vi "rs3 Set All Advanced5.vi"(0 "Set Color Corr":bool=TRUE, 1 "Depth Presets":T2(ring), 2 "Color Presets":T1(ring), 7 "error in (no error)":errorcluster, 8 "device in":u64=370866768, 10 "ST_CensusEnable":cluster{"uDiameter":u32, "vDiameter":u32}={"uDiameter"=9, "vDiameter"=9}, 12 "ST_AE_Control":cluster{"meanIntensitySetpoint":u32}={"meanIntensitySetpoint"=400}, 16 "Depth Table":T3={"depthUnits, um"=1000, "depthClampMin"=0, "depthClampMax"=65535, "disparityMultiplier"=0, "disparityShift"=0}, 17 "ST RAU vector":T9={"minWest"=1, "minEast"=1, "minWEsum"=1, "minNorth"=1, "minSouth"=1, "minNSSum"=1, "uStrink"=1, "vShrink"=1}, 19 "ST Color Control":T8, 20 "depth control":T4={"plusIncrement"=10, "MinusDecrement"=10, "deepSeaMedianThreshold"=528, "scoreThreshA"=10, "scoreThreshB"=1023, "textureDifferenceThreshold"=0, "textureCountThreshold"=0, "deepSeaSecondPeakThreshold"=27, "deepSeaNeighborThreshold"=20, "IrAgreeThreshold"=70}, 21 "STColorCorrection":T11={"colorCorrection 1"=0.54785156, "colorCorrection 2"=0.32910156, "colorCorrection 3"=0.8222656, "colorCorrection 4"=0.109375, "colorCorrection 5"=-0.40527344, "colorCorrection 6"=-1.5253906, "colorCorrection 7"=0.95703125, "colorCorrection 8"=0.89160156, "colorCorrection 9"=0.7675781, "colorCorrection 10"=-0.4794922, "colorCorrection 11"=0.047851562, "colorCorrection 12"=-0.2705078}, 22 "HDAD":T12={"lambdaCensus"=26.0, "lambdaAD"=2100.0, "ignoreSAD"=0}, 23 "ST RSM":T10={"rsmBypass"=0, "diffThresh"=7.0, "sloRauDiffThresh"=3.0, "removeThresh"=33}, 24 "ST SLO Penalty":T5={"sloK1Penalty"=44, "sloK2Penalty"=502, "sloK1PenaltyMod1"=23, "sloK2PenaltyMod1"=237, "sloK1PenaltyMod2"=219, "sloK2PenaltyMod2"=113}, 25 "ST SLO Threshold":T6={"SLOdiffThresholdRed"=300, "SLODiffThresholdGreen"=300, "SLODiffThresholdBlue"=300}, 26 "ST Rau Threshold":T7={"rauDiffThresholdRed"=600, "rauDiffThresholdGreen"=600, "rauDiffThresholdBlue"=600}) -> (14 "Set advanced error":string, 18 "Dev out":u64=370866768, 27 "error out":errorcluster)   [LabVIEW 2018, in "libRealSense3.lvlib"]
doc: "The RealSense D4xx cameras are based on a stereo algorithm that has been accelerated as a fixed-function inside an ASIC. There are many parameters that affect the calculation of the depth. The basic task is to solve the correspondance problem - i.e. figure out which patches in the left image match up to those in the right image by doing a search along an epipolar line (x-axis). The x-axis difference for each object point is known as the disparity. \n\nIn general depth can be estimated for most points in the scene, but some points will have a very low confidence because 1. they are may be occluded (not seen by both imagers), or 2. have very little texture on them which will lead to an ambiquity (ex. when looking at a completely uniform white wall it, there are no best correspondances).\n\nThis VI allows you to set the many parameters that affect the algorith, as well as the color reproduction. \nNote that the color correction matrix will NOT have any effect on the depth calculations."
uses:
  libRealSense3.lvlib
panel:
  # "RS3 Set All Advanced 5"
  # "(C) 2017 Intel Corp.,  AGJ"
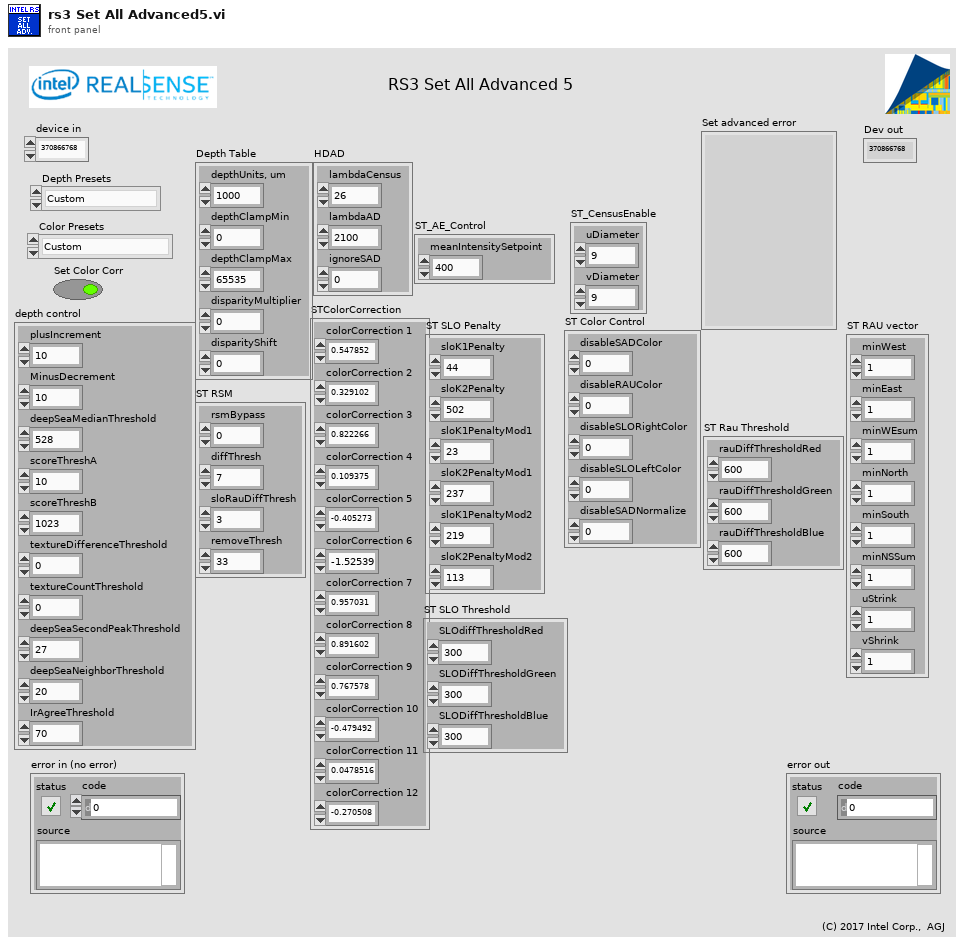
[diagram p1: front panel]
types:
  T1 = enum16{"Custom", "RS400 (DS5p)", "RS400 (DS5p) 2", "RS400 (DS5p) 3", "RS400 (DS5p) 4", "RS400 (DS5p) 5", "RS410 (DS5a)", "RS410 (DS5a) 2", "DS410 (DS5a) 3", "DS410 (DS5a) 4", "DS410+IR", "DS5LR", "DS5LR-2", "DS5LR no pattern", "RS410 Remove IR", "RS410 Remove IR 2", "DS5micro", "D435"}
  T2 = enum16{"Custom", "Original", "New Depth 1", "New Depth 2", "Depth Active 1", "Active 3D Scan", "Active Short A", "Active Short C", "Face", "Face2", "Best Box", "High Density", "Medium Density", "High Accuracy", "Hand", "Short Range", "Flat wall", "Load .JSON", "Load .JSON2"}
  T3 = cluster{"depthUnits, um":u32, "depthClampMin":u32, "depthClampMax":u32, "disparityMultiplier":u32, "disparityShift":u32}
  T4 = cluster{"plusIncrement":u32, "MinusDecrement":u32, "deepSeaMedianThreshold":u32, "scoreThreshA":u32, "scoreThreshB":u32, "textureDifferenceThreshold":u32, "textureCountThreshold":u32, "deepSeaSecondPeakThreshold":u32, "deepSeaNeighborThreshold":u32, "IrAgreeThreshold":u32}
  T5 = cluster{"sloK1Penalty":u32, "sloK2Penalty":u32, "sloK1PenaltyMod1":u32, "sloK2PenaltyMod1":u32, "sloK1PenaltyMod2":u32, "sloK2PenaltyMod2":u32}
  T6 = cluster{"SLOdiffThresholdRed":u32, "SLODiffThresholdGreen":u32, "SLODiffThresholdBlue":u32}
  T7 = cluster{"rauDiffThresholdRed":u32, "rauDiffThresholdGreen":u32, "rauDiffThresholdBlue":u32}
  T8 = cluster{"disableSADColor":u32, "disableRAUColor":u32, "disableSLORightColor":u32, "disableSLOLeftColor":u32, "disableSADNormalize":u32}
  T9 = cluster{"minWest":u32, "minEast":u32, "minWEsum":u32, "minNorth":u32, "minSouth":u32, "minNSSum":u32, "uStrink":u32, "vShrink":u32}
  T10 = cluster{"rsmBypass":u32, "diffThresh":sgl, "sloRauDiffThresh":sgl, "removeThresh":u32}
  T11 = cluster{"colorCorrection 1":sgl, "colorCorrection 2":sgl, "colorCorrection 3":sgl, "colorCorrection 4":sgl, "colorCorrection 5":sgl, "colorCorrection 6":sgl, "colorCorrection 7":sgl, "colorCorrection 8":sgl, "colorCorrection 9":sgl, "colorCorrection 10":sgl, "colorCorrection 11":sgl, "colorCorrection 12":sgl}
  T12 = cluster{"lambdaCensus":sgl, "lambdaAD":sgl, "ignoreSAD":u32}
  T13 = cluster{"rsmBypass (56)":u32, "diffThresh (57)":sgl, "sloRauDiffThresh(58)":sgl, "removeThresh(59)":u32}
  T14 = cluster{"depth control":cluster{"plusIncrement":u32, "MinusDecrement":u32, "deepSeaMedianThreshold":u32, "scoreThreshA":u32, "scoreThreshB":u32, "textureDifferenceThreshold":u32, "textureCountThreshold":u32, "deepSeaSecondPeakThreshold":u32, "deepSeaNeighborThreshold":u32, "IrAgreeThreshold":u32}, "STColorCorrection output":cluster{"colorCorrection 1":sgl, "colorCorrection 2":sgl, "colorCorrection 3":sgl, "colorCorrection 4":sgl, "colorCorrection 5":sgl, "colorCorrection 6":sgl, "colorCorrection 7":sgl, "colorCorrection 8":sgl, "colorCorrection 9":sgl, "colorCorrection 10":sgl, "colorCorrection 11":sgl, "colorCorrection 12":sgl}, "HDAD":cluster{"lambdaCensus":sgl, "lambdaAD":sgl, "ignoreSAD":u32}, "ST RSM":cluster{"rsmBypass":u32, "diffThresh":sgl, "sloRauDiffThresh":sgl, "removeThresh":u32}, "ST SLO Penalty":cluster{"sloK1Penalty":u32, "sloK2Penalty":u32, "sloK1PenaltyMod1":u32, "sloK2PenaltyMod1":u32, "sloK1PenaltyMod2":u32, "sloK2PenaltyMod2":u32}, "ST SLO Threshold":cluster{"SLOdiffThresholdRed":u32, "SLODiffThresholdGreen":u32, "SLODiffThresholdBlue":u32}, "ST Rau Threshold":cluster{"rauDiffThresholdRed":u32, "rauDiffThresholdGreen":u32, "rauDiffThresholdBlue":u32}, "ST Color Control":cluster{"disableSADColor":u32, "disableRAUColor":u32, "disableSLORightColor":u32, "disableSLOLeftColor":u32, "disableSADNormalize":u32}, "ST RAU vector":cluster{"minWest":u32, "minEast":u32, "minWEsum":u32, "minNorth":u32, "minSouth":u32, "minNSSum":u32, "uStrink":u32, "vShrink":u32}, "Depth Table":cluster{"depthUnits, um":u32, "depthClampMin":u32, "depthClampMax":u32, "disparityMultiplier":u32, "disparityShift":u32}, "ST_AE_Control":cluster{"meanIntensitySetpoint":u32}, "ST_CensusEnable":cluster{"uDiameter":u32, "vDiameter":u32}}
  T15 = cluster{"depthUnits, um":u32, "depthClampMin":u32, "depthClampMax":u32, "disparityMultiplier":u32, "disparityShift(0-127)":u32}
  T16 = cluster{"minWest (60)":u32, "minEast (61)":u32, "minWEsum (62)":u32, "minNorth (63)":u32, "minSouth (64)":u32, "minNSSum(65)":u32, "uStrink (66)":u32, "vShrink (67)":u32}
  T17 = cluster{"rauDiffThreshRed(73)":u32, "rauDiffThreshGreen(74)":u32, "rauDiffThreshBlue(75)":u32}
  T18 = cluster{"sloK1Penalty (79)":u32, "sloK2Penalty (80)":u32, "sloK1PenaltyMod1(81)":u32, "sloK2PenaltyMod1(82)":u32, "sloK1PenaltyMod2(83)":u32, "sloK2PenaltyMod2(84)":u32}
  T19 = cluster{"SLOdiffThreshRed(76)":u32, "SLODiffThreshGreen(77)":u32, "SLODiffThreshBlue(78)":u32}
  T20 = cluster{"disableSADColor(68)":u32, "disableRAUColor(69)":u32, "disableSLORightColor(70)":u32, "disableSLOLeftColor(71)":u32, "disableSADNormalize(72)":u32}
  T21 = cluster{"plusIncrement (47)":u32, "MinusDecrement (46)":u32, "deepSeaMedianThreshold (48)":u32, "scoreThreshA(49)":u32, "scoreThreshB (50)":u32, "textureDifferenceThreshold (52)":u32, "textureCountThreshold (51)":u32, "deepSea2ndPeakThresh.(53)":u32, "deepSeaNeighborThresh.(54)":u32, "LRAgreeThreshold (55)":u32}
  T22 = cluster{"plusIncrement (47)":u32, "MinusDecrement (46)":u32, "deepSeaMedianThreshold (48)":u32, "scoreThreshA(49)":u32, "scoreThreshB (50)":u32, "textureDifferenceThreshold (52)":u32, "textureCountThreshold (51)":u32, "deepSea2ndPeakThresh.(53)":u32, "deepSeaNeighborThresh.(54)":u32, "IrAgreeThreshold (55)":u32}
  T23 = cluster{"DS5p- 1":sgl, "colorCorrection 2":sgl, "colorCorrection 3":sgl, "colorCorrection 4":sgl, "colorCorrection 5":sgl, "colorCorrection 6":sgl, "colorCorrection 7":sgl, "colorCorrection 8":sgl, "colorCorrection 9":sgl, "colorCorrection 10":sgl, "colorCorrection 11":sgl, "colorCorrection 12":sgl}
  T24 = cluster{"Color 0":dbl, "Color 1":dbl, "Color 2":dbl, "Color 3":dbl, "Color 4":dbl, "Color 5":dbl, "Color 6":dbl, "Color 7":dbl, "Color 8":dbl, "Color 9":dbl, "Color 10":dbl, "Color 11":dbl}
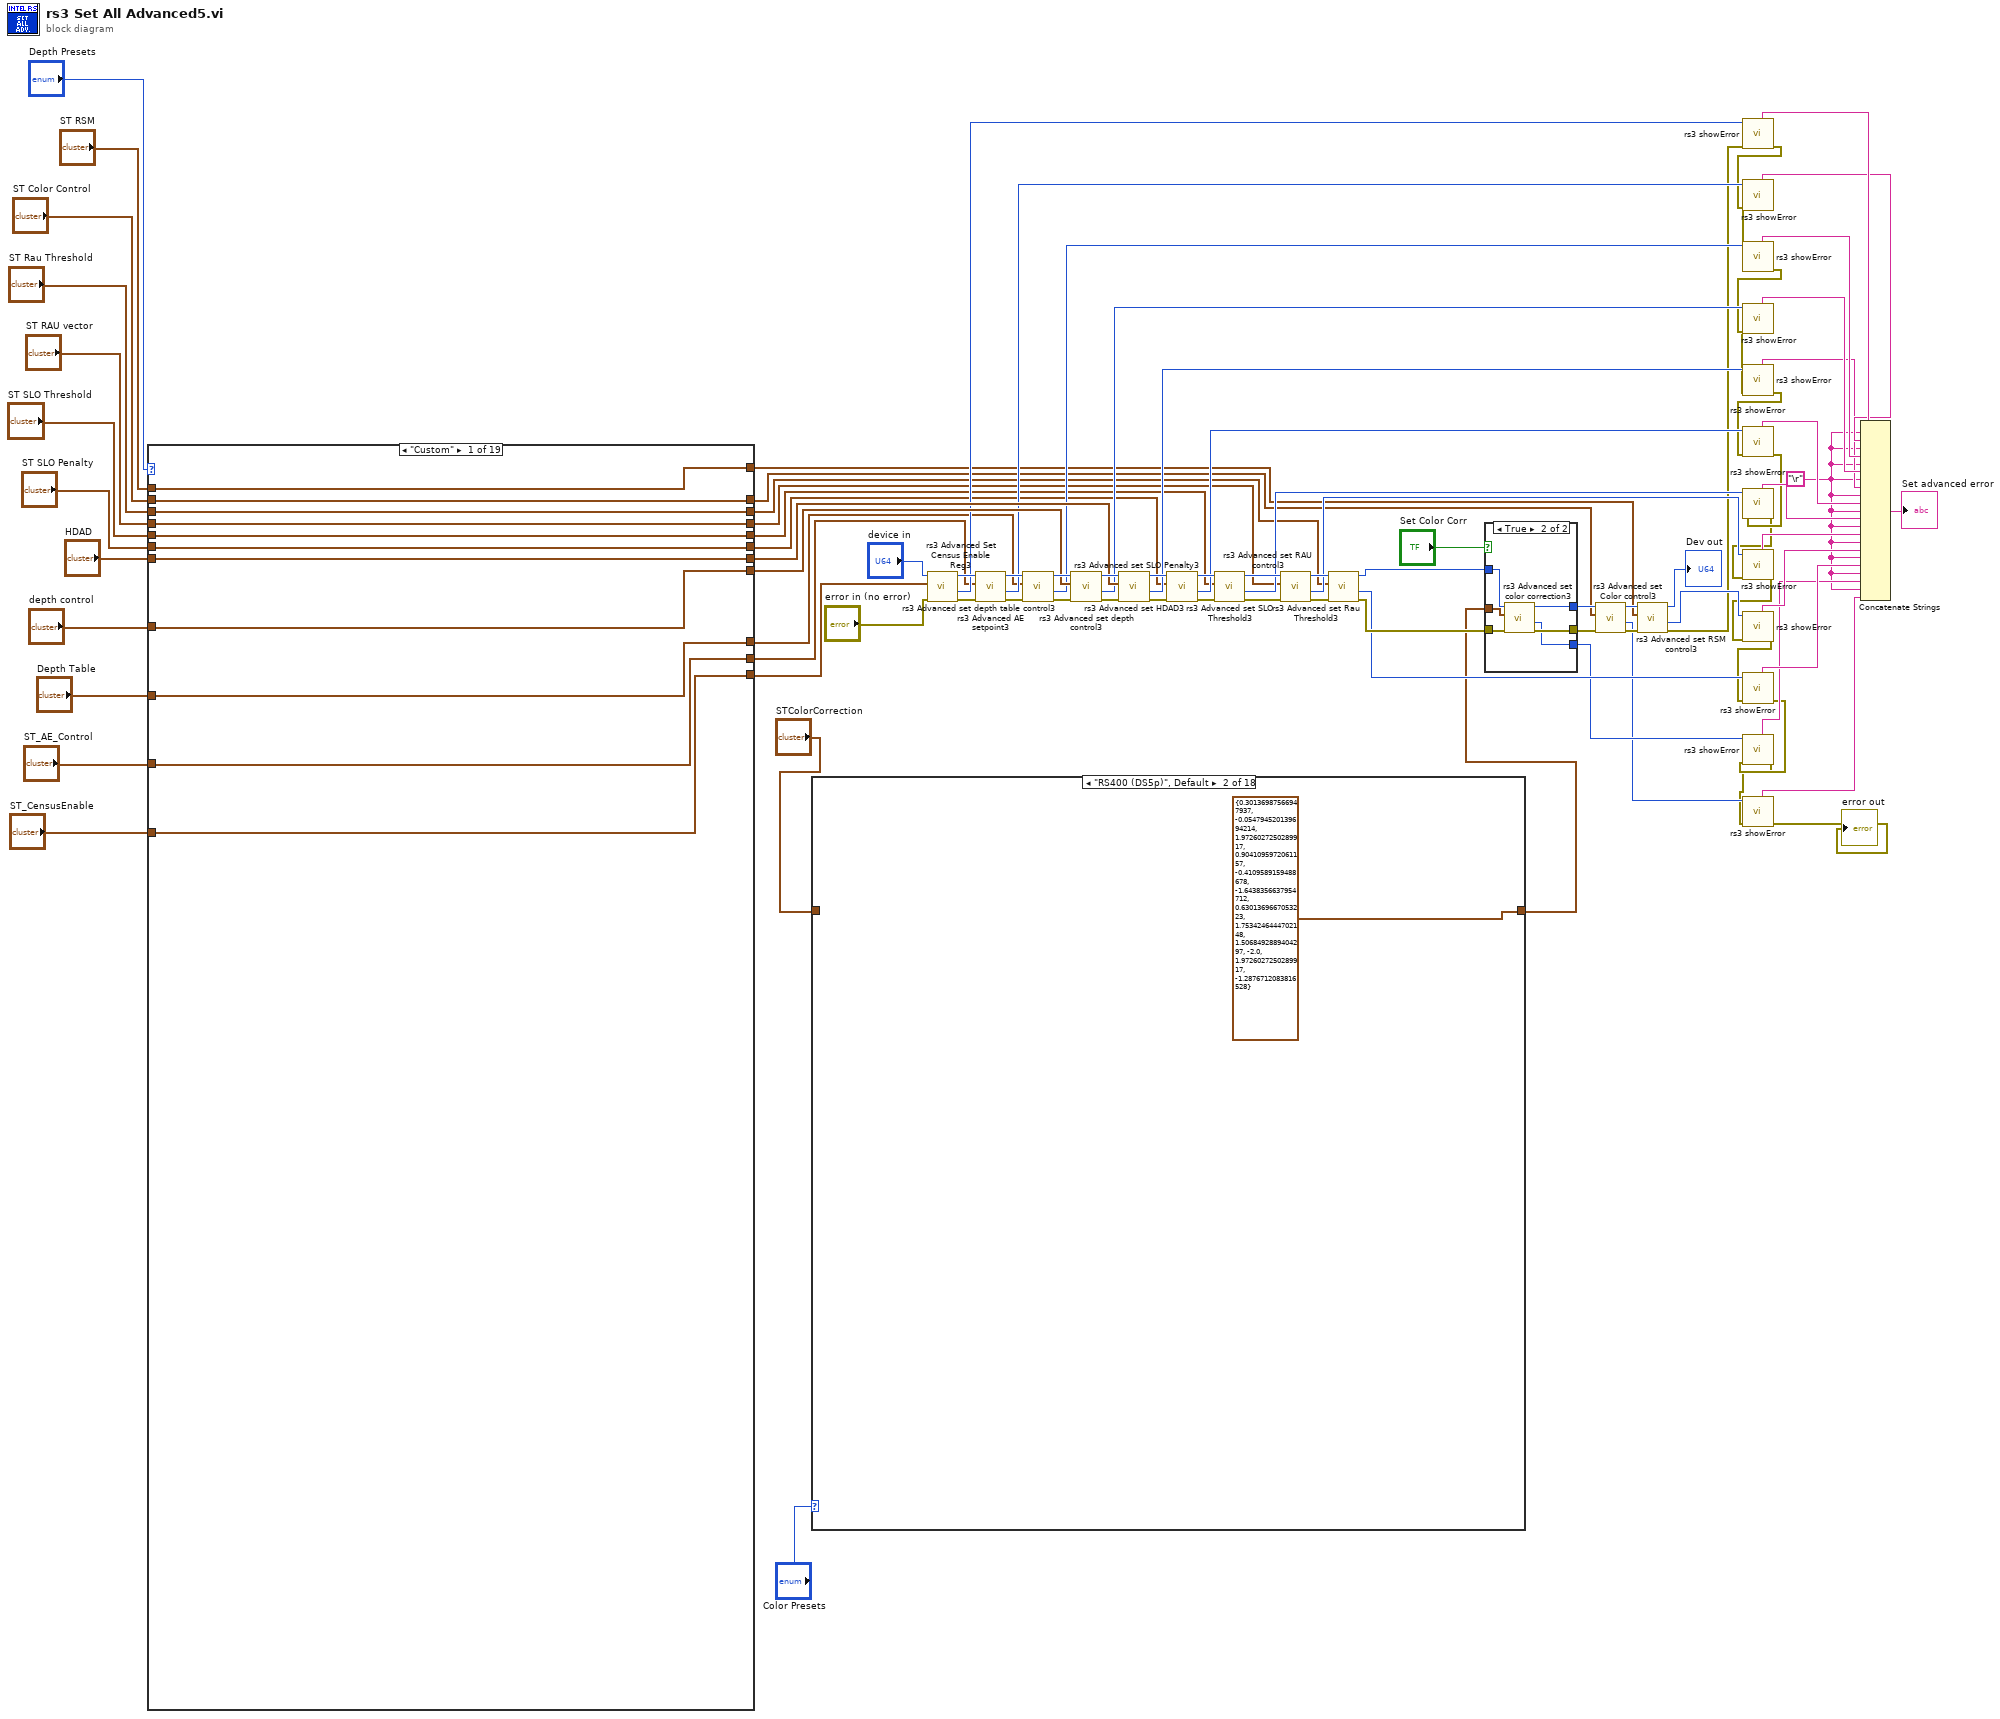
[diagram p0: block diagram]
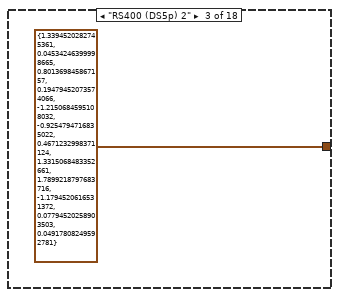
[diagram p3: hidden frame]
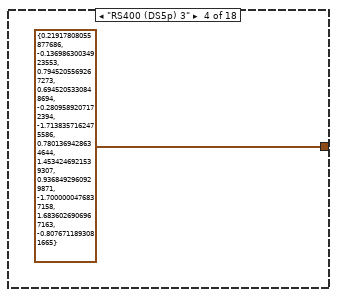
[diagram p4: hidden frame]
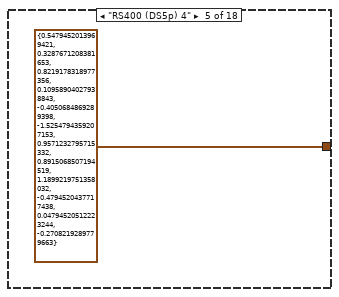
[diagram p5: hidden frame]
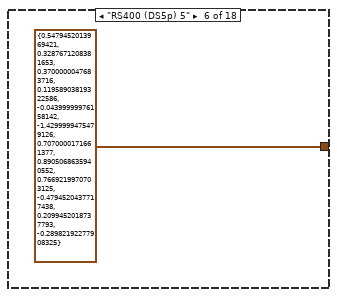
[diagram p6: hidden frame]
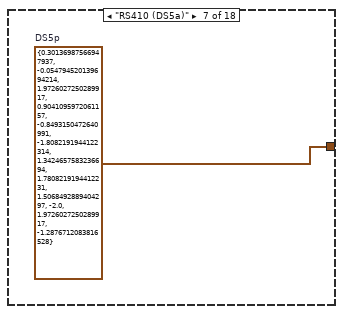
[diagram p7: hidden frame]
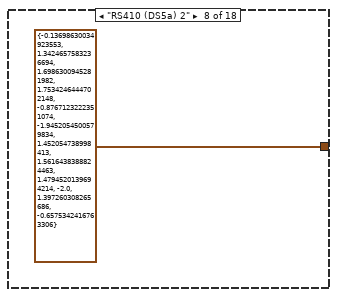
[diagram p8: hidden frame]
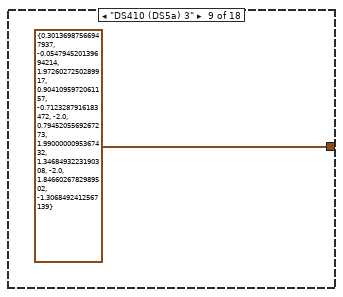
[diagram p9: hidden frame]
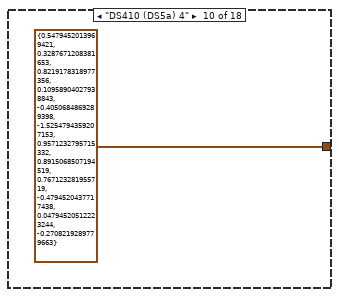
[diagram p10: hidden frame]
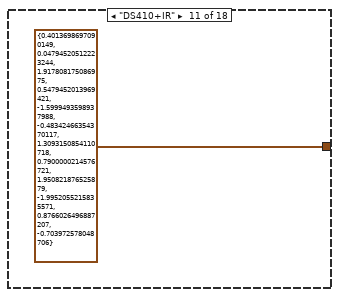
[diagram p11: hidden frame]
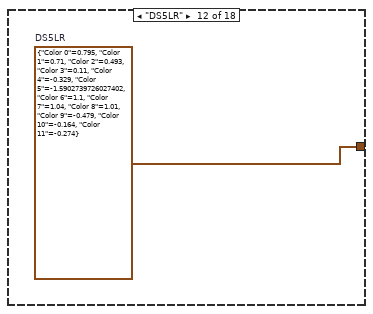
[diagram p12: hidden frame]
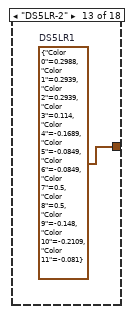
[diagram p13: hidden frame]
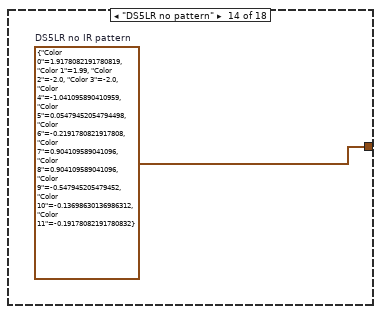
[diagram p14: hidden frame]
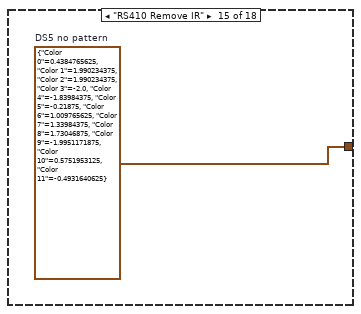
[diagram p15: hidden frame]
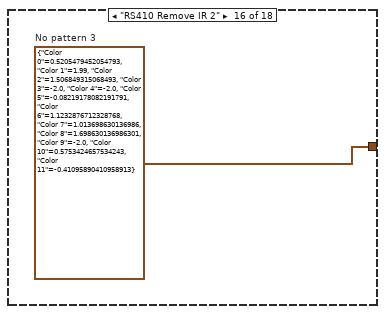
[diagram p16: hidden frame]
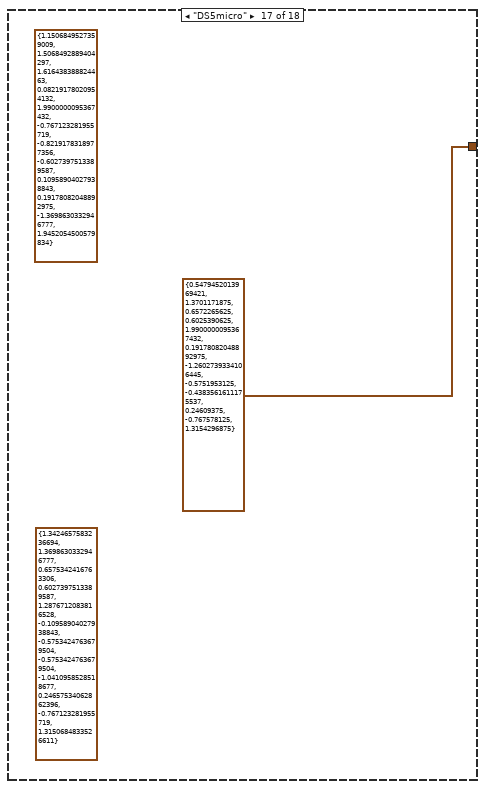
[diagram p17: hidden frame]
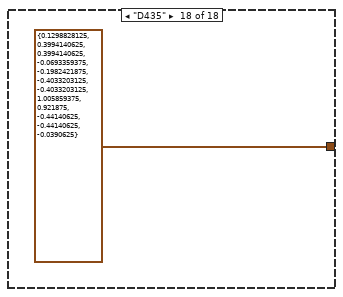
[diagram p18: hidden frame]
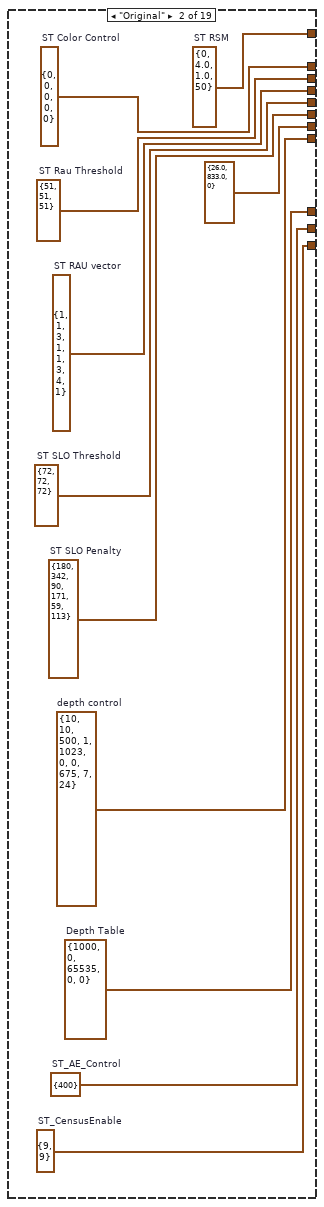
[diagram p19: hidden frame]
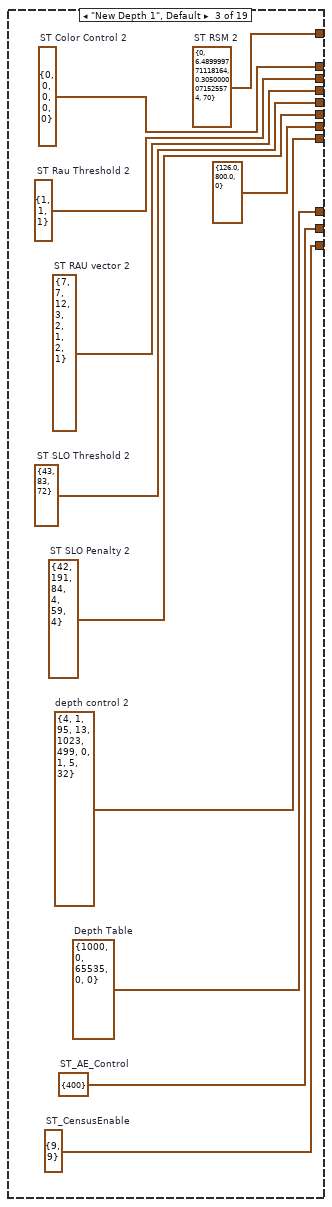
[diagram p20: hidden frame]
diagram:
  w36 = "\r"
  n1 = case shown="\"Custom\"" "Depth Presets" {
    tunnel: [w102 w112 w124 w135 w146 w150 w161 w172 w188 w198 w209 w216 w229 w241 w253 w265 w277 w292 w306] -> w63
    tunnel: [w96 w111 w123 w134 w145 T13 {"rsmBypass (56)"=0, "diffThresh (57)"=1.0367311, "sloRauDiffThresh(58)"=151.0, "removeThresh(59)"=1} ("ST RSM 2") w168 w179 w190 w195 w206 w221 w234 w246 w258 w270 w282 w294 w308] -> w25
    tunnel: [w97 w106 w122 w133 w144 w157 w167 w178 w189 w196 w207 w223 w236 w248 w260 w272 w284 w291 w305] -> w27
    tunnel: [w98 w107 w121 w132 w143 w156 w166 w177 w186 w197 w208 w219 w232 w244 w256 w268 w280 w295 w309] -> w28
    tunnel: [w95 w110 w120 w131 w142 w155 w165 w176 w185 w199 w210 w215 w228 w240 w252 w264 w276 w298 w312] -> w23
    tunnel: [w99 w109 w119 w130 w141 w154 w164 w175 w183 w200 w211 w214 w227 w239 w251 w263 w275 w297 w311] -> w30
    tunnel: [w100 w108 w118 w129 w140 w153 w163 w174 w187 w201 w212 w213 w226 w238 w250 w262 w274 w296 w310] -> w33
    tunnel: [w101 T12 {"lambdaCensus"=26.0, "lambdaAD"=833.0, "ignoreSAD"=0} ("HDAD 2") T12 {"lambdaCensus"=126.0, "lambdaAD"=800.0, "ignoreSAD"=0} ("HDAD 2") T12 {"lambdaCensus"=200.0, "lambdaAD"=1900.0, "ignoreSAD"=0} ("HDAD 2") T12 {"lambdaCensus"=216.0, "lambdaAD"=1400.0, "ignoreSAD"=0} ("HDAD 2") T12 {"lambdaCensus"=26.0, "lambdaAD"=833.0, "ignoreSAD"=0} ("HDAD 2") T12 {"lambdaCensus"=100.0, "lambdaAD"=1600.0, "ignoreSAD"=0} ("HDAD 2") w173 w184 T12 {"lambdaCensus"=26.0, "lambdaAD"=2100.0, "ignoreSAD"=0} ("HDAD*") T12 {"lambdaCensus"=15.0, "lambdaAD"=618.0, "ignoreSAD"=0} ("HDAD*") w222 w235 w247 w259 w271 w283 w293 w307] -> w61
    tunnel: [w93 w103 w114 w125 w136 w147 w158 w170 w180 w191 w202 w217 w230 w242 w254 w266 w278 w285 w301] -> w19
    tunnel: [w94 w104 w115 w126 w137 w148 w159 w169 w181 w192 w203 w218 w231 w243 w255 w267 w279 w286 w300] -> w21
    tunnel: [w92 w105 w116 w127 w138 w149 w160 w171 w182 w193 w204 w220 w233 w245 w257 w269 w281 w287 w299] -> w17
    tunnel: "depth control" -> [w102 _ _ _ _ _ _ _ _ _ _ _ _ _ _ _ _ _ _]
    tunnel: "HDAD" -> [w101 _ _ _ _ _ _ _ _ _ _ _ _ _ _ _ _ _ _]
    tunnel: "ST SLO Penalty" -> [w100 _ _ _ _ _ _ _ _ _ _ _ _ _ _ _ _ _ _]
    tunnel: "ST SLO Threshold" -> [w99 _ _ _ _ _ _ _ _ _ _ _ _ _ _ _ _ _ _]
    tunnel: "ST RAU vector" -> [w97 _ _ _ _ _ _ _ _ _ _ _ _ _ _ _ _ _ _]
    tunnel: "ST Rau Threshold" -> [w98 _ _ _ _ _ _ _ _ _ _ _ _ _ _ _ _ _ _]
    tunnel: "ST RSM" -> [w96 _ _ _ _ _ _ _ _ _ _ _ _ _ _ _ _ _ _]
    tunnel: "ST Color Control" -> [w95 _ _ _ _ _ _ _ _ _ _ _ _ _ _ _ _ _ _]
    tunnel: "ST_CensusEnable" -> [w94 _ _ _ _ _ _ _ _ _ _ _ _ _ _ _ _ _ _]
    tunnel: "ST_AE_Control" -> [w93 _ _ _ _ _ _ _ _ _ _ _ _ _ _ _ _ _ _]
    tunnel: "Depth Table" -> [w92 _ _ _ _ _ _ _ _ _ _ _ _ _ _ _ _ _ _]
    frame "Custom" {
    }
    frame "Original" {
      w104 = cluster{"uDiameter":u32, "vDiameter":u32} {"uDiameter"=9, "vDiameter"=9}  # ST_CensusEnable
      w105 = T15 {"depthUnits, um"=1000, "depthClampMin"=0, "depthClampMax"=65535, "disparityMultiplier"=0, "disparityShift(0-127)"=0}  # Depth Table
      w103 = cluster{"meanIntensitySetpoint":u32} {"meanIntensitySetpoint"=400}  # ST_AE_Control
      w106 = T16 {"minWest (60)"=1, "minEast (61)"=1, "minWEsum (62)"=3, "minNorth (63)"=1, "minSouth (64)"=1, "minNSSum(65)"=3, "uStrink (66)"=4, "vShrink (67)"=1}  # ST RAU vector
      w107 = T17 {"rauDiffThreshRed(73)"=51, "rauDiffThreshGreen(74)"=51, "rauDiffThreshBlue(75)"=51}  # ST Rau Threshold
      w108 = T18 {"sloK1Penalty (79)"=180, "sloK2Penalty (80)"=342, "sloK1PenaltyMod1(81)"=90, "sloK2PenaltyMod1(82)"=171, "sloK1PenaltyMod2(83)"=59, "sloK2PenaltyMod2(84)"=113}  # ST SLO Penalty
      w109 = T19 {"SLOdiffThreshRed(76)"=72, "SLODiffThreshGreen(77)"=72, "SLODiffThreshBlue(78)"=72}  # ST SLO Threshold
      w110 = T20 {"disableSADColor(68)"=0, "disableRAUColor(69)"=0, "disableSLORightColor(70)"=0, "disableSLOLeftColor(71)"=0, "disableSADNormalize(72)"=0}  # ST Color Control
      w111 = T13 {"rsmBypass (56)"=0, "diffThresh (57)"=4.0, "sloRauDiffThresh(58)"=1.0, "removeThresh(59)"=50}  # ST RSM
      w112 = T21 {"plusIncrement (47)"=10, "MinusDecrement (46)"=10, "deepSeaMedianThreshold (48)"=500, "scoreThreshA(49)"=1, "scoreThreshB (50)"=1023, "textureDifferenceThreshold (52)"=0, "textureCountThreshold (51)"=0, "deepSea2ndPeakThresh.(53)"=675, "deepSeaNeighborThresh.(54)"=7, "LRAgreeThreshold (55)"=24}  # depth control
    }
    frame "New Depth 1", Default {
      w115 = cluster{"uDiameter":u32, "vDiameter":u32} {"uDiameter"=9, "vDiameter"=9}  # ST_CensusEnable
      w116 = T15 {"depthUnits, um"=1000, "depthClampMin"=0, "depthClampMax"=65535, "disparityMultiplier"=0, "disparityShift(0-127)"=0}  # Depth Table
      w114 = cluster{"meanIntensitySetpoint":u32} {"meanIntensitySetpoint"=400}  # ST_AE_Control
      w118 = T18 {"sloK1Penalty (79)"=42, "sloK2Penalty (80)"=191, "sloK1PenaltyMod1(81)"=84, "sloK2PenaltyMod1(82)"=4, "sloK1PenaltyMod2(83)"=59, "sloK2PenaltyMod2(84)"=4}  # ST SLO Penalty 2
      w119 = T19 {"SLOdiffThreshRed(76)"=43, "SLODiffThreshGreen(77)"=83, "SLODiffThreshBlue(78)"=72}  # ST SLO Threshold 2
      w120 = T20 {"disableSADColor(68)"=0, "disableRAUColor(69)"=0, "disableSLORightColor(70)"=0, "disableSLOLeftColor(71)"=0, "disableSADNormalize(72)"=0}  # ST Color Control 2
      w121 = T17 {"rauDiffThreshRed(73)"=1, "rauDiffThreshGreen(74)"=1, "rauDiffThreshBlue(75)"=1}  # ST Rau Threshold 2
      w122 = T16 {"minWest (60)"=7, "minEast (61)"=7, "minWEsum (62)"=12, "minNorth (63)"=3, "minSouth (64)"=2, "minNSSum(65)"=1, "uStrink (66)"=2, "vShrink (67)"=1}  # ST RAU vector 2
      w123 = T13 {"rsmBypass (56)"=0, "diffThresh (57)"=6.49, "sloRauDiffThresh(58)"=0.305, "removeThresh(59)"=70}  # ST RSM 2
      w124 = T22 {"plusIncrement (47)"=4, "MinusDecrement (46)"=1, "deepSeaMedianThreshold (48)"=95, "scoreThreshA(49)"=13, "scoreThreshB (50)"=1023, "textureDifferenceThreshold (52)"=499, "textureCountThreshold (51)"=0, "deepSea2ndPeakThresh.(53)"=1, "deepSeaNeighborThresh.(54)"=5, "IrAgreeThreshold (55)"=32}  # depth control 2
    }
    frame "New Depth 2" {
      w126 = cluster{"uDiameter":u32, "vDiameter":u32} {"uDiameter"=9, "vDiameter"=9}  # ST_CensusEnable
      w127 = T15 {"depthUnits, um"=1000, "depthClampMin"=0, "depthClampMax"=65535, "disparityMultiplier"=0, "disparityShift(0-127)"=0}  # Depth Table
      w125 = cluster{"meanIntensitySetpoint":u32} {"meanIntensitySetpoint"=400}  # ST_AE_Control
      w129 = T18 {"sloK1Penalty (79)"=42, "sloK2Penalty (80)"=191, "sloK1PenaltyMod1(81)"=84, "sloK2PenaltyMod1(82)"=4, "sloK1PenaltyMod2(83)"=59, "sloK2PenaltyMod2(84)"=4}  # ST SLO Penalty 2
      w130 = T19 {"SLOdiffThreshRed(76)"=100, "SLODiffThreshGreen(77)"=100, "SLODiffThreshBlue(78)"=100}  # ST SLO Threshold 2
      w131 = T20 {"disableSADColor(68)"=0, "disableRAUColor(69)"=0, "disableSLORightColor(70)"=0, "disableSLOLeftColor(71)"=0, "disableSADNormalize(72)"=0}  # ST Color Control 2
      w132 = T17 {"rauDiffThreshRed(73)"=50, "rauDiffThreshGreen(74)"=50, "rauDiffThreshBlue(75)"=50}  # ST Rau Threshold 2
      w133 = T16 {"minWest (60)"=1, "minEast (61)"=1, "minWEsum (62)"=9, "minNorth (63)"=3, "minSouth (64)"=2, "minNSSum(65)"=1, "uStrink (66)"=2, "vShrink (67)"=1}  # ST RAU vector 2
      w134 = T13 {"rsmBypass (56)"=0, "diffThresh (57)"=6.49, "sloRauDiffThresh(58)"=0.305, "removeThresh(59)"=50}  # ST RSM 2
      w135 = T22 {"plusIncrement (47)"=4, "MinusDecrement (46)"=1, "deepSeaMedianThreshold (48)"=95, "scoreThreshA(49)"=13, "scoreThreshB (50)"=1023, "textureDifferenceThreshold (52)"=499, "textureCountThreshold (51)"=0, "deepSea2ndPeakThresh.(53)"=1, "deepSeaNeighborThresh.(54)"=5, "IrAgreeThreshold (55)"=200}  # depth control 2
    }
    frame "Depth Active 1" {
      w137 = cluster{"uDiameter":u32, "vDiameter":u32} {"uDiameter"=9, "vDiameter"=9}  # ST_CensusEnable
      w138 = T15 {"depthUnits, um"=1000, "depthClampMin"=0, "depthClampMax"=65535, "disparityMultiplier"=0, "disparityShift(0-127)"=0}  # Depth Table
      w136 = cluster{"meanIntensitySetpoint":u32} {"meanIntensitySetpoint"=400}  # ST_AE_Control
      w140 = T18 {"sloK1Penalty (79)"=10, "sloK2Penalty (80)"=60, "sloK1PenaltyMod1(81)"=84, "sloK2PenaltyMod1(82)"=56, "sloK1PenaltyMod2(83)"=59, "sloK2PenaltyMod2(84)"=4}  # ST SLO Penalty 2
      w141 = T19 {"SLOdiffThreshRed(76)"=200, "SLODiffThreshGreen(77)"=200, "SLODiffThreshBlue(78)"=200}  # ST SLO Threshold 2
      w142 = T20 {"disableSADColor(68)"=0, "disableRAUColor(69)"=0, "disableSLORightColor(70)"=0, "disableSLOLeftColor(71)"=0, "disableSADNormalize(72)"=0}  # ST Color Control 2
      w143 = T17 {"rauDiffThreshRed(73)"=70, "rauDiffThreshGreen(74)"=70, "rauDiffThreshBlue(75)"=70}  # ST Rau Threshold 2
      w144 = T16 {"minWest (60)"=7, "minEast (61)"=7, "minWEsum (62)"=12, "minNorth (63)"=3, "minSouth (64)"=2, "minNSSum(65)"=1, "uStrink (66)"=2, "vShrink (67)"=1}  # ST RAU vector 2
      w145 = T13 {"rsmBypass (56)"=0, "diffThresh (57)"=6.49, "sloRauDiffThresh(58)"=0.305, "removeThresh(59)"=60}  # ST RSM 2
      w146 = T22 {"plusIncrement (47)"=4, "MinusDecrement (46)"=1, "deepSeaMedianThreshold (48)"=95, "scoreThreshA(49)"=13, "scoreThreshB (50)"=1023, "textureDifferenceThreshold (52)"=499, "textureCountThreshold (51)"=0, "deepSea2ndPeakThresh.(53)"=1, "deepSeaNeighborThresh.(54)"=5, "IrAgreeThreshold (55)"=82}  # depth control 2
    }
    frame "Active 3D Scan" {
      w148 = cluster{"uDiameter":u32, "vDiameter":u32} {"uDiameter"=9, "vDiameter"=9}  # ST_CensusEnable
      w149 = T15 {"depthUnits, um"=1000, "depthClampMin"=0, "depthClampMax"=65535, "disparityMultiplier"=0, "disparityShift(0-127)"=0}  # Depth Table
      w147 = cluster{"meanIntensitySetpoint":u32} {"meanIntensitySetpoint"=400}  # ST_AE_Control
      w150 = T22 {"plusIncrement (47)"=19, "MinusDecrement (46)"=4, "deepSeaMedianThreshold (48)"=554, "scoreThreshA(49)"=1, "scoreThreshB (50)"=632, "textureDifferenceThreshold (52)"=0, "textureCountThreshold (51)"=31, "deepSea2ndPeakThresh.(53)"=665, "deepSeaNeighborThresh.(54)"=126, "IrAgreeThreshold (55)"=11}  # depth control 2
      w153 = T18 {"sloK1Penalty (79)"=93, "sloK2Penalty (80)"=473, "sloK1PenaltyMod1(81)"=70, "sloK2PenaltyMod1(82)"=123, "sloK1PenaltyMod2(83)"=92, "sloK2PenaltyMod2(84)"=409}  # ST SLO Penalty 2
      w154 = T19 {"SLOdiffThreshRed(76)"=46, "SLODiffThreshGreen(77)"=442, "SLODiffThreshBlue(78)"=105}  # ST SLO Threshold 2
      w155 = T20 {"disableSADColor(68)"=0, "disableRAUColor(69)"=0, "disableSLORightColor(70)"=0, "disableSLOLeftColor(71)"=0, "disableSADNormalize(72)"=0}  # ST Color Control 2
      w156 = T17 {"rauDiffThreshRed(73)"=46, "rauDiffThreshGreen(74)"=442, "rauDiffThreshBlue(75)"=105}  # ST Rau Threshold 2
      w157 = T16 {"minWest (60)"=5, "minEast (61)"=7, "minWEsum (62)"=12, "minNorth (63)"=1, "minSouth (64)"=3, "minNSSum(65)"=7, "uStrink (66)"=4, "vShrink (67)"=1}  # ST RAU vector 2
    }
    frame "Active Short A" {
      w159 = cluster{"uDiameter":u32, "vDiameter":u32} {"uDiameter"=3, "vDiameter"=3}  # ST_CensusEnable
      w160 = T15 {"depthUnits, um"=200, "depthClampMin"=0, "depthClampMax"=65535, "disparityMultiplier"=0, "disparityShift(0-127)"=0}  # Depth Table
      w158 = cluster{"meanIntensitySetpoint":u32} {"meanIntensitySetpoint"=400}  # ST_AE_Control
      w161 = T22 {"plusIncrement (47)"=7, "MinusDecrement (46)"=1, "deepSeaMedianThreshold (48)"=140, "scoreThreshA(49)"=10, "scoreThreshB (50)"=1023, "textureDifferenceThreshold (52)"=499, "textureCountThreshold (51)"=0, "deepSea2ndPeakThresh.(53)"=1, "deepSeaNeighborThresh.(54)"=5, "IrAgreeThreshold (55)"=80}  # depth control 2
      w163 = T18 {"sloK1Penalty (79)"=5, "sloK2Penalty (80)"=30, "sloK1PenaltyMod1(81)"=11, "sloK2PenaltyMod1(82)"=50, "sloK1PenaltyMod2(83)"=56, "sloK2PenaltyMod2(84)"=15}  # ST SLO Penalty 2
      w164 = T19 {"SLOdiffThreshRed(76)"=200, "SLODiffThreshGreen(77)"=200, "SLODiffThreshBlue(78)"=200}  # ST SLO Threshold 2
      w165 = T20 {"disableSADColor(68)"=0, "disableRAUColor(69)"=0, "disableSLORightColor(70)"=0, "disableSLOLeftColor(71)"=0, "disableSADNormalize(72)"=0}  # ST Color Control 2
      w166 = T17 {"rauDiffThreshRed(73)"=200, "rauDiffThreshGreen(74)"=200, "rauDiffThreshBlue(75)"=200}  # ST Rau Threshold 2
      w167 = T16 {"minWest (60)"=3, "minEast (61)"=3, "minWEsum (62)"=13, "minNorth (63)"=1, "minSouth (64)"=1, "minNSSum(65)"=1, "uStrink (66)"=4, "vShrink (67)"=4}  # ST RAU vector 2
      w168 = T13 {"rsmBypass (56)"=0, "diffThresh (57)"=7.5, "sloRauDiffThresh(58)"=0.9, "removeThresh(59)"=72}  # ST RSM 2
    }
    frame "Active Short C" {
      w169 = cluster{"uDiameter":u32, "vDiameter":u32} {"uDiameter"=3, "vDiameter"=3}  # ST_CensusEnable
      w171 = T15 {"depthUnits, um"=200, "depthClampMin"=0, "depthClampMax"=65535, "disparityMultiplier"=0, "disparityShift(0-127)"=0}  # Depth Table
      w170 = cluster{"meanIntensitySetpoint":u32} {"meanIntensitySetpoint"=400}  # ST_AE_Control
      w172 = T22 {"plusIncrement (47)"=10, "MinusDecrement (46)"=10, "deepSeaMedianThreshold (48)"=415, "scoreThreshA(49)"=1, "scoreThreshB (50)"=1023, "textureDifferenceThreshold (52)"=0, "textureCountThreshold (51)"=14, "deepSea2ndPeakThresh.(53)"=56, "deepSeaNeighborThresh.(54)"=108, "IrAgreeThreshold (55)"=8}  # depth control 2
      w173 = T12 {"lambdaCensus"=26.0, "lambdaAD"=958.0, "ignoreSAD"=0}  # HDAD 2
      w174 = T18 {"sloK1Penalty (79)"=203, "sloK2Penalty (80)"=342, "sloK1PenaltyMod1(81)"=109, "sloK2PenaltyMod1(82)"=502, "sloK1PenaltyMod2(83)"=209, "sloK2PenaltyMod2(84)"=14}  # ST SLO Penalty 2
      w175 = T19 {"SLOdiffThreshRed(76)"=889, "SLODiffThreshGreen(77)"=69, "SLODiffThreshBlue(78)"=189}  # ST SLO Threshold 2
      w176 = T20 {"disableSADColor(68)"=0, "disableRAUColor(69)"=0, "disableSLORightColor(70)"=0, "disableSLOLeftColor(71)"=0, "disableSADNormalize(72)"=0}  # ST Color Control 2
      w177 = T17 {"rauDiffThreshRed(73)"=298, "rauDiffThreshGreen(74)"=95, "rauDiffThreshBlue(75)"=675}  # ST Rau Threshold 2
      w178 = T16 {"minWest (60)"=1, "minEast (61)"=1, "minWEsum (62)"=3, "minNorth (63)"=1, "minSouth (64)"=1, "minNSSum(65)"=3, "uStrink (66)"=3, "vShrink (67)"=1}  # ST RAU vector 2
      w179 = T13 {"rsmBypass (56)"=0, "diffThresh (57)"=5.386, "sloRauDiffThresh(58)"=0.9687, "removeThresh(59)"=88}  # ST RSM 2
    }
    frame "Face" {
      w181 = cluster{"uDiameter":u32, "vDiameter":u32} {"uDiameter"=9, "vDiameter"=9}  # ST_CensusEnable
      w182 = T15 {"depthUnits, um"=1000, "depthClampMin"=0, "depthClampMax"=65535, "disparityMultiplier"=0, "disparityShift(0-127)"=0}  # Depth Table
      w180 = cluster{"meanIntensitySetpoint":u32} {"meanIntensitySetpoint"=800}  # ST_AE_Control
      w184 = T12 {"lambdaCensus"=26.0, "lambdaAD"=2100.0, "ignoreSAD"=0}  # HDAD*
      w183 = T19 {"SLOdiffThreshRed(76)"=300, "SLODiffThreshGreen(77)"=300, "SLODiffThreshBlue(78)"=300}  # ST SLO Threshold
      w185 = T20 {"disableSADColor(68)"=0, "disableRAUColor(69)"=0, "disableSLORightColor(70)"=0, "disableSLOLeftColor(71)"=0, "disableSADNormalize(72)"=0}  # ST Color Control
      w186 = T17 {"rauDiffThreshRed(73)"=600, "rauDiffThreshGreen(74)"=600, "rauDiffThreshBlue(75)"=600}  # ST Rau Threshold
      w187 = T18 {"sloK1Penalty (79)"=44, "sloK2Penalty (80)"=502, "sloK1PenaltyMod1(81)"=23, "sloK2PenaltyMod1(82)"=237, "sloK1PenaltyMod2(83)"=219, "sloK2PenaltyMod2(84)"=113}  # ST SLO Penalty
      w188 = T21 {"plusIncrement (47)"=10, "MinusDecrement (46)"=10, "deepSeaMedianThreshold (48)"=528, "scoreThreshA(49)"=10, "scoreThreshB (50)"=1023, "textureDifferenceThreshold (52)"=0, "textureCountThreshold (51)"=0, "deepSea2ndPeakThresh.(53)"=27, "deepSeaNeighborThresh.(54)"=20, "LRAgreeThreshold (55)"=70}  # depth control
      w189 = T16 {"minWest (60)"=1, "minEast (61)"=1, "minWEsum (62)"=1, "minNorth (63)"=1, "minSouth (64)"=1, "minNSSum(65)"=1, "uStrink (66)"=1, "vShrink (67)"=1}  # ST RAU vector
      w190 = T13 {"rsmBypass (56)"=0, "diffThresh (57)"=7.0, "sloRauDiffThresh(58)"=3.0, "removeThresh(59)"=33}  # ST RSM
    }
    frame "Face2" {
      w192 = cluster{"uDiameter":u32, "vDiameter":u32} {"uDiameter"=9, "vDiameter"=9}  # ST_CensusEnable
      w193 = T15 {"depthUnits, um"=1000, "depthClampMin"=0, "depthClampMax"=65535, "disparityMultiplier"=0, "disparityShift(0-127)"=0}  # Depth Table
      w191 = cluster{"meanIntensitySetpoint":u32} {"meanIntensitySetpoint"=800}  # ST_AE_Control
      w195 = T13 {"rsmBypass (56)"=0, "diffThresh (57)"=1.21875, "sloRauDiffThresh(58)"=0.28125, "removeThresh(59)"=83}  # ST RSM
      w196 = T16 {"minWest (60)"=3, "minEast (61)"=2, "minWEsum (62)"=7, "minNorth (63)"=1, "minSouth (64)"=3, "minNSSum(65)"=6, "uStrink (66)"=4, "vShrink (67)"=0}  # ST RAU vector
      w197 = T17 {"rauDiffThreshRed(73)"=18, "rauDiffThreshGreen(74)"=113, "rauDiffThreshBlue(75)"=586}  # ST Rau Threshold
      w198 = T21 {"plusIncrement (47)"=10, "MinusDecrement (46)"=10, "deepSeaMedianThreshold (48)"=528, "scoreThreshA(49)"=10, "scoreThreshB (50)"=1023, "textureDifferenceThreshold (52)"=0, "textureCountThreshold (51)"=0, "deepSea2ndPeakThresh.(53)"=27, "deepSeaNeighborThresh.(54)"=20, "LRAgreeThreshold (55)"=70}  # depth control
      w199 = T20 {"disableSADColor(68)"=0, "disableRAUColor(69)"=0, "disableSLORightColor(70)"=0, "disableSLOLeftColor(71)"=0, "disableSADNormalize(72)"=0}  # ST Color Control
      w200 = T19 {"SLOdiffThreshRed(76)"=279, "SLODiffThreshGreen(77)"=200, "SLODiffThreshBlue(78)"=8}  # ST SLO Threshold
      w201 = T18 {"sloK1Penalty (79)"=55, "sloK2Penalty (80)"=235, "sloK1PenaltyMod1(81)"=326, "sloK2PenaltyMod1(82)"=506, "sloK1PenaltyMod2(83)"=134, "sloK2PenaltyMod2(84)"=206}  # ST SLO Penalty
    }
    frame "Best Box" {
      w203 = cluster{"uDiameter":u32, "vDiameter":u32} {"uDiameter"=9, "vDiameter"=9}  # ST_CensusEnable
      w204 = T15 {"depthUnits, um"=1000, "depthClampMin"=0, "depthClampMax"=65535, "disparityMultiplier"=0, "disparityShift(0-127)"=0}  # Depth Table
      w202 = cluster{"meanIntensitySetpoint":u32} {"meanIntensitySetpoint"=400}  # ST_AE_Control
      w206 = T13 {"rsmBypass (56)"=0, "diffThresh (57)"=1.21875, "sloRauDiffThresh(58)"=0.28125, "removeThresh(59)"=83}  # ST RSM
      w207 = T16 {"minWest (60)"=3, "minEast (61)"=2, "minWEsum (62)"=7, "minNorth (63)"=1, "minSouth (64)"=3, "minNSSum(65)"=6, "uStrink (66)"=4, "vShrink (67)"=0}  # ST RAU vector
      w208 = T17 {"rauDiffThreshRed(73)"=18, "rauDiffThreshGreen(74)"=113, "rauDiffThreshBlue(75)"=586}  # ST Rau Threshold
      w209 = T21 {"plusIncrement (47)"=10, "MinusDecrement (46)"=10, "deepSeaMedianThreshold (48)"=528, "scoreThreshA(49)"=10, "scoreThreshB (50)"=1023, "textureDifferenceThreshold (52)"=0, "textureCountThreshold (51)"=0, "deepSea2ndPeakThresh.(53)"=27, "deepSeaNeighborThresh.(54)"=20, "LRAgreeThreshold (55)"=70}  # depth control
      w210 = T20 {"disableSADColor(68)"=0, "disableRAUColor(69)"=0, "disableSLORightColor(70)"=0, "disableSLOLeftColor(71)"=0, "disableSADNormalize(72)"=0}  # ST Color Control
      w211 = T19 {"SLOdiffThreshRed(76)"=279, "SLODiffThreshGreen(77)"=200, "SLODiffThreshBlue(78)"=8}  # ST SLO Threshold
      w212 = T18 {"sloK1Penalty (79)"=55, "sloK2Penalty (80)"=235, "sloK1PenaltyMod1(81)"=326, "sloK2PenaltyMod1(82)"=506, "sloK1PenaltyMod2(83)"=134, "sloK2PenaltyMod2(84)"=206}  # ST SLO Penalty
    }
    frame "High Density" {
      n2 = Unbundle By Name(T14 {"depth control"={"plusIncrement"=21, "MinusDecrement"=6, "deepSeaMedianThreshold"=789, "scoreThreshA"=96, "scoreThreshB"=1443, "textureDifferenceThreshold"=2466, "textureCountThreshold"=0, "deepSeaSecondPeakThreshold"=222, "deepSeaNeighborThreshold"=12, "IrAgreeThreshold"=18}, "STColorCorrection output"={"colorCorrection 1"=0.54785156, "colorCorrection 2"=0.32910156, "colorCorrection 3"=0.8222656, "colorCorrection 4"=0.109375, "colorCorrection 5"=-0.40527344, "colorCorrection 6"=-1.5253906, "colorCorrection 7"=0.95703125, "colorCorrection 8"=0.89160156, "colorCorrection 9"=0.7675781, "colorCorrection 10"=-0.4794922, "colorCorrection 11"=0.047851562, "colorCorrection 12"=-0.2705078}, "HDAD"={"lambdaCensus"=15.0, "lambdaAD"=618.0, "ignoreSAD"=0}, "ST RSM"={"rsmBypass"=0, "diffThresh"=1.21875, "sloRauDiffThresh"=0.28125, "removeThresh"=82}, "ST SLO Penalty"={"sloK1Penalty"=55, "sloK2Penalty"=235, "sloK1PenaltyMod1"=326, "sloK2PenaltyMod1"=506, "sloK1PenaltyMod2"=134, "sloK2PenaltyMod2"=206}, "ST SLO Threshold"={"SLOdiffThresholdRed"=279, "SLODiffThresholdGreen"=200, "SLODiffThresholdBlue"=8}, "ST Rau Threshold"={"rauDiffThresholdRed"=18, "rauDiffThresholdGreen"=585, "rauDiffThresholdBlue"=112}, "ST Color Control"={"disableSADColor"=0, "disableRAUColor"=0, "disableSLORightColor"=0, "disableSLOLeftColor"=0, "disableSADNormalize"=0}, "ST RAU vector"={"minWest"=3, "minEast"=2, "minWEsum"=7, "minNorth"=1, "minSouth"=3, "minNSSum"=6, "uStrink"=4, "vShrink"=0}, "Depth Table"={"depthUnits, um"=1000, "depthClampMin"=0, "depthClampMax"=65535, "disparityMultiplier"=0, "disparityShift"=0}, "ST_AE_Control"={"meanIntensitySetpoint"=800}, "ST_CensusEnable"={"uDiameter"=9, "vDiameter"=9}} ("depth settings 2")) -> ("depth control"=w216:T4, "HDAD"=w222:T12, "ST RSM"=w221:T10, "ST SLO Penalty"=w213:T5, "ST SLO Threshold"=w214:T6, "ST Rau Threshold"=w219:T7, "ST Color Control"=w215:T8, "ST RAU vector"=w223:T9, "Depth Table"=w220:T3, "ST_AE_Control"=w217:cluster{"meanIntensitySetpoint":u32}, "ST_CensusEnable"=w218:cluster{"uDiameter":u32, "vDiameter":u32})  [unwired: 1 out]
    }
    frame "Medium Density" {
      n3 = Unbundle By Name(T14 {"depth control"={"plusIncrement"=3, "MinusDecrement"=23, "deepSeaMedianThreshold"=1021, "scoreThreshA"=54, "scoreThreshB"=887, "textureDifferenceThreshold"=0, "textureCountThreshold"=0, "deepSeaSecondPeakThreshold"=600, "deepSeaNeighborThreshold"=97, "IrAgreeThreshold"=19}, "STColorCorrection output"={"colorCorrection 1"=0.4013672, "colorCorrection 2"=0.047851562, "colorCorrection 3"=1.9179688, "colorCorrection 4"=0.54785156, "colorCorrection 5"=-1.5996094, "colorCorrection 6"=-0.48339844, "colorCorrection 7"=1.3095703, "colorCorrection 8"=0.79003906, "colorCorrection 9"=1.9511719, "colorCorrection 10"=-1.9951172, "colorCorrection 11"=0.8769531, "colorCorrection 12"=-0.70410156}, "HDAD"={"lambdaCensus"=26.0, "lambdaAD"=935.0, "ignoreSAD"=0}, "ST RSM"={"rsmBypass"=0, "diffThresh"=1.8125, "sloRauDiffThresh"=1.0, "removeThresh"=81}, "ST SLO Penalty"={"sloK1Penalty"=132, "sloK2Penalty"=342, "sloK1PenaltyMod1"=77, "sloK2PenaltyMod1"=390, "sloK1PenaltyMod2"=234, "sloK2PenaltyMod2"=151}, "ST SLO Threshold"={"SLOdiffThresholdRed"=896, "SLODiffThresholdGreen"=259, "SLODiffThresholdBlue"=16}, "ST Rau Threshold"={"rauDiffThresholdRed"=186, "rauDiffThresholdGreen"=723, "rauDiffThresholdBlue"=14}, "ST Color Control"={"disableSADColor"=0, "disableRAUColor"=0, "disableSLORightColor"=1, "disableSLOLeftColor"=0, "disableSADNormalize"=0}, "ST RAU vector"={"minWest"=5, "minEast"=3, "minWEsum"=11, "minNorth"=1, "minSouth"=3, "minNSSum"=6, "uStrink"=3, "vShrink"=1}, "Depth Table"={"depthUnits, um"=1000, "depthClampMin"=0, "depthClampMax"=65535, "disparityMultiplier"=0, "disparityShift"=0}, "ST_AE_Control"={"meanIntensitySetpoint"=800}, "ST_CensusEnable"={"uDiameter"=9, "vDiameter"=9}} ("depth settings 2")) -> ("depth control"=w229:T4, "HDAD"=w235:T12, "ST RSM"=w234:T10, "ST SLO Penalty"=w226:T5, "ST SLO Threshold"=w227:T6, "ST Rau Threshold"=w232:T7, "ST Color Control"=w228:T8, "ST RAU vector"=w236:T9, "Depth Table"=w233:T3, "ST_AE_Control"=w230:cluster{"meanIntensitySetpoint":u32}, "ST_CensusEnable"=w231:cluster{"uDiameter":u32, "vDiameter":u32})  [unwired: 1 out]
    }
    frame "High Accuracy" {
      n4 = Unbundle By Name(T14 {"depth control"={"plusIncrement"=2, "MinusDecrement"=25, "deepSeaMedianThreshold"=796, "scoreThreshA"=4, "scoreThreshB"=2893, "textureDifferenceThreshold"=1722, "textureCountThreshold"=0, "deepSeaSecondPeakThreshold"=647, "deepSeaNeighborThreshold"=108, "IrAgreeThreshold"=10}, "STColorCorrection output"={"colorCorrection 1"=0.4013672, "colorCorrection 2"=0.047851562, "colorCorrection 3"=1.9179688, "colorCorrection 4"=0.54785156, "colorCorrection 5"=-1.5996094, "colorCorrection 6"=-0.48339844, "colorCorrection 7"=1.3095703, "colorCorrection 8"=0.79003906, "colorCorrection 9"=1.9511719, "colorCorrection 10"=-1.9951172, "colorCorrection 11"=0.8769531, "colorCorrection 12"=-0.70410156}, "HDAD"={"lambdaCensus"=26.0, "lambdaAD"=935.0, "ignoreSAD"=0}, "ST RSM"={"rsmBypass"=0, "diffThresh"=1.65625, "sloRauDiffThresh"=0.71875, "removeThresh"=137}, "ST SLO Penalty"={"sloK1Penalty"=155, "sloK2Penalty"=190, "sloK1PenaltyMod1"=160, "sloK2PenaltyMod1"=507, "sloK1PenaltyMod2"=59, "sloK2PenaltyMod2"=493}, "ST SLO Threshold"={"SLOdiffThresholdRed"=30, "SLODiffThresholdGreen"=15, "SLODiffThresholdBlue"=13}, "ST Rau Threshold"={"rauDiffThresholdRed"=1007, "rauDiffThresholdGreen"=578, "rauDiffThresholdBlue"=803}, "ST Color Control"={"disableSADColor"=0, "disableRAUColor"=0, "disableSLORightColor"=1, "disableSLOLeftColor"=0, "disableSADNormalize"=0}, "ST RAU vector"={"minWest"=2, "minEast"=6, "minWEsum"=12, "minNorth"=3, "minSouth"=2, "minNSSum"=7, "uStrink"=3, "vShrink"=0}, "Depth Table"={"depthUnits, um"=1000, "depthClampMin"=0, "depthClampMax"=65535, "disparityMultiplier"=0, "disparityShift"=0}, "ST_AE_Control"={"meanIntensitySetpoint"=800}, "ST_CensusEnable"={"uDiameter"=9, "vDiameter"=9}} ("depth settings 2")) -> ("depth control"=w241:T4, "HDAD"=w247:T12, "ST RSM"=w246:T10, "ST SLO Penalty"=w238:T5, "ST SLO Threshold"=w239:T6, "ST Rau Threshold"=w244:T7, "ST Color Control"=w240:T8, "ST RAU vector"=w248:T9, "Depth Table"=w245:T3, "ST_AE_Control"=w242:cluster{"meanIntensitySetpoint":u32}, "ST_CensusEnable"=w243:cluster{"uDiameter":u32, "vDiameter":u32})  [unwired: 1 out]
    }
    frame "Hand" {
      n5 = Unbundle By Name(T14 {"depth control"={"plusIncrement"=3, "MinusDecrement"=20, "deepSeaMedianThreshold"=240, "scoreThreshA"=24, "scoreThreshB"=791, "textureDifferenceThreshold"=783, "textureCountThreshold"=0, "deepSeaSecondPeakThreshold"=31, "deepSeaNeighborThreshold"=110, "IrAgreeThreshold"=20}, "STColorCorrection output"={"colorCorrection 1"=0.4013672, "colorCorrection 2"=0.047851562, "colorCorrection 3"=1.9179688, "colorCorrection 4"=0.54785156, "colorCorrection 5"=-1.5996094, "colorCorrection 6"=-0.48339844, "colorCorrection 7"=1.3095703, "colorCorrection 8"=0.79003906, "colorCorrection 9"=1.9511719, "colorCorrection 10"=-1.9951172, "colorCorrection 11"=0.8769531, "colorCorrection 12"=-0.70410156}, "HDAD"={"lambdaCensus"=7.0, "lambdaAD"=1001.0, "ignoreSAD"=0}, "ST RSM"={"rsmBypass"=0, "diffThresh"=3.8125, "sloRauDiffThresh"=0.46875, "removeThresh"=94}, "ST SLO Penalty"={"sloK1Penalty"=63, "sloK2Penalty"=45, "sloK1PenaltyMod1"=14, "sloK2PenaltyMod1"=21, "sloK1PenaltyMod2"=119, "sloK2PenaltyMod2"=12}, "ST SLO Threshold"={"SLOdiffThresholdRed"=618, "SLODiffThresholdGreen"=244, "SLODiffThresholdBlue"=130}, "ST Rau Threshold"={"rauDiffThresholdRed"=141, "rauDiffThresholdGreen"=74, "rauDiffThresholdBlue"=50}, "ST Color Control"={"disableSADColor"=0, "disableRAUColor"=0, "disableSLORightColor"=1, "disableSLOLeftColor"=0, "disableSADNormalize"=0}, "ST RAU vector"={"minWest"=1, "minEast"=3, "minWEsum"=14, "minNorth"=1, "minSouth"=3, "minNSSum"=4, "uStrink"=3, "vShrink"=1}, "Depth Table"={"depthUnits, um"=1000, "depthClampMin"=0, "depthClampMax"=65535, "disparityMultiplier"=0, "disparityShift"=0}, "ST_AE_Control"={"meanIntensitySetpoint"=800}, "ST_CensusEnable"={"uDiameter"=9, "vDiameter"=9}} ("depth settings 2")) -> ("depth control"=w253:T4, "HDAD"=w259:T12, "ST RSM"=w258:T10, "ST SLO Penalty"=w250:T5, "ST SLO Threshold"=w251:T6, "ST Rau Threshold"=w256:T7, "ST Color Control"=w252:T8, "ST RAU vector"=w260:T9, "Depth Table"=w257:T3, "ST_AE_Control"=w254:cluster{"meanIntensitySetpoint":u32}, "ST_CensusEnable"=w255:cluster{"uDiameter":u32, "vDiameter":u32})  [unwired: 1 out]
    }
    frame "Short Range" {
      n6 = Unbundle By Name(T14 {"depth control"={"plusIncrement"=10, "MinusDecrement"=10, "deepSeaMedianThreshold"=528, "scoreThreshA"=10, "scoreThreshB"=1023, "textureDifferenceThreshold"=0, "textureCountThreshold"=0, "deepSeaSecondPeakThreshold"=27, "deepSeaNeighborThreshold"=20, "IrAgreeThreshold"=70}, "STColorCorrection output"={"colorCorrection 1"=0.4013672, "colorCorrection 2"=0.047851562, "colorCorrection 3"=1.9179688, "colorCorrection 4"=0.54785156, "colorCorrection 5"=-1.5996094, "colorCorrection 6"=-0.48339844, "colorCorrection 7"=1.3095703, "colorCorrection 8"=0.79003906, "colorCorrection 9"=1.9511719, "colorCorrection 10"=-1.9951172, "colorCorrection 11"=0.8769531, "colorCorrection 12"=-0.70410156}, "HDAD"={"lambdaCensus"=26.0, "lambdaAD"=935.0, "ignoreSAD"=0}, "ST RSM"={"rsmBypass"=0, "diffThresh"=7.0, "sloRauDiffThresh"=3.0, "removeThresh"=32}, "ST SLO Penalty"={"sloK1Penalty"=44, "sloK2Penalty"=502, "sloK1PenaltyMod1"=23, "sloK2PenaltyMod1"=237, "sloK1PenaltyMod2"=219, "sloK2PenaltyMod2"=113}, "ST SLO Threshold"={"SLOdiffThresholdRed"=300, "SLODiffThresholdGreen"=300, "SLODiffThresholdBlue"=300}, "ST Rau Threshold"={"rauDiffThresholdRed"=599, "rauDiffThresholdGreen"=599, "rauDiffThresholdBlue"=599}, "ST Color Control"={"disableSADColor"=0, "disableRAUColor"=0, "disableSLORightColor"=0, "disableSLOLeftColor"=0, "disableSADNormalize"=0}, "ST RAU vector"={"minWest"=1, "minEast"=1, "minWEsum"=1, "minNorth"=1, "minSouth"=1, "minNSSum"=1, "uStrink"=1, "vShrink"=1}, "Depth Table"={"depthUnits, um"=1000, "depthClampMin"=0, "depthClampMax"=65535, "disparityMultiplier"=0, "disparityShift"=0}, "ST_AE_Control"={"meanIntensitySetpoint"=800}, "ST_CensusEnable"={"uDiameter"=9, "vDiameter"=9}} ("depth settings 2")) -> ("depth control"=w265:T4, "HDAD"=w271:T12, "ST RSM"=w270:T10, "ST SLO Penalty"=w262:T5, "ST SLO Threshold"=w263:T6, "ST Rau Threshold"=w268:T7, "ST Color Control"=w264:T8, "ST RAU vector"=w272:T9, "Depth Table"=w269:T3, "ST_AE_Control"=w266:cluster{"meanIntensitySetpoint":u32}, "ST_CensusEnable"=w267:cluster{"uDiameter":u32, "vDiameter":u32})  [unwired: 1 out]
    }
    frame "Flat wall" {
      # "AndersDepth4"
      n7 = Unbundle By Name(T14 {"depth control"={"plusIncrement"=10, "MinusDecrement"=10, "deepSeaMedianThreshold"=528, "scoreThreshA"=10, "scoreThreshB"=1023, "textureDifferenceThreshold"=0, "textureCountThreshold"=0, "deepSeaSecondPeakThreshold"=27, "deepSeaNeighborThreshold"=20, "IrAgreeThreshold"=70}, "STColorCorrection output"={"colorCorrection 1"=0.4013672, "colorCorrection 2"=0.047851562, "colorCorrection 3"=1.9179688, "colorCorrection 4"=0.54785156, "colorCorrection 5"=-1.5996094, "colorCorrection 6"=-0.48339844, "colorCorrection 7"=1.3095703, "colorCorrection 8"=0.79003906, "colorCorrection 9"=1.9511719, "colorCorrection 10"=-1.9951172, "colorCorrection 11"=0.8769531, "colorCorrection 12"=-0.70410156}, "HDAD"={"lambdaCensus"=26.0, "lambdaAD"=935.0, "ignoreSAD"=0}, "ST RSM"={"rsmBypass"=0, "diffThresh"=7.0, "sloRauDiffThresh"=3.0, "removeThresh"=32}, "ST SLO Penalty"={"sloK1Penalty"=44, "sloK2Penalty"=502, "sloK1PenaltyMod1"=23, "sloK2PenaltyMod1"=237, "sloK1PenaltyMod2"=219, "sloK2PenaltyMod2"=113}, "ST SLO Threshold"={"SLOdiffThresholdRed"=300, "SLODiffThresholdGreen"=300, "SLODiffThresholdBlue"=300}, "ST Rau Threshold"={"rauDiffThresholdRed"=599, "rauDiffThresholdGreen"=599, "rauDiffThresholdBlue"=599}, "ST Color Control"={"disableSADColor"=0, "disableRAUColor"=0, "disableSLORightColor"=0, "disableSLOLeftColor"=0, "disableSADNormalize"=0}, "ST RAU vector"={"minWest"=1, "minEast"=1, "minWEsum"=1, "minNorth"=1, "minSouth"=1, "minNSSum"=1, "uStrink"=1, "vShrink"=1}, "Depth Table"={"depthUnits, um"=1000, "depthClampMin"=0, "depthClampMax"=65535, "disparityMultiplier"=0, "disparityShift"=0}, "ST_AE_Control"={"meanIntensitySetpoint"=800}, "ST_CensusEnable"={"uDiameter"=9, "vDiameter"=9}} ("depth settings 2")) -> ("depth control"=w277:T4, "HDAD"=w283:T12, "ST RSM"=w282:T10, "ST SLO Penalty"=w274:T5, "ST SLO Threshold"=w275:T6, "ST Rau Threshold"=w280:T7, "ST Color Control"=w276:T8, "ST RAU vector"=w284:T9, "Depth Table"=w281:T3, "ST_AE_Control"=w278:cluster{"meanIntensitySetpoint":u32}, "ST_CensusEnable"=w279:cluster{"uDiameter":u32, "vDiameter":u32})  [unwired: 1 out]
    }
    frame "Load .JSON" {
      w286 = cluster{"uDiameter":u32, "vDiameter":u32} {"uDiameter"=9, "vDiameter"=9}  # ST_CensusEnable
      w287 = T15 {"depthUnits, um"=1000, "depthClampMin"=0, "depthClampMax"=65535, "disparityMultiplier"=0, "disparityShift(0-127)"=0}  # Depth Table
      w285 = cluster{"meanIntensitySetpoint":u32} {"meanIntensitySetpoint"=400}  # ST_AE_Control
      n8 = call "File Dialog"("prompt"="Load .JSON file", "pattern (all files)"="*.json") -> ("selected path"=w290:path)  [unwired: 10 in, 3 out]
      n9 = call "rs3_ReadDepthPreference3.vi"("file (use dialog)"=w290) -> ("HDAD 2*"=w293:T12, "ST Color Control 2"=w298:T20, "depth control 2"=w292:T22, "ST RSM 2"=w294:T13, "ST SLO Penalty 2"=w296:T18, "ST SLO Threshold 2"=w297:T19, "ST Rau Threshold 2"=w295:T17, "ST RAU vector 2"=w291:T16)  [unwired: 5 in, 2 out]
    }
    frame "Load .JSON2" {
      n10 = call "File Dialog2"("prompt"="Load .JSON file", "pattern (all files)"="*.json") -> ("selected path"=w304:path)  [unwired: 10 in, 3 out]
      n11 = call "rs3_ReadDepthPreference4.vi"("file (use dialog)"=w304) -> ("HDAD 2*"=w307:T12, "ST_AE_Control"=w301:cluster{"meanIntensitySetpoint":u32}, "ST Color Control 2"=w312:T20, "depth control 2"=w306:T22, "ST RSM 2"=w308:T13, "Depth Table"=w299:T15, "ST SLO Penalty 2"=w310:T18, "ST_CensusEnable"=w300:cluster{"uDiameter":u32, "vDiameter":u32}, "ST SLO Threshold 2"=w311:T19, "ST Rau Threshold 2"=w309:T17, "ST RAU vector 2"=w305:T16)  [unwired: 2 in, 2 out]
    }
  }
  n12 = case shown="\"RS400 (DS5p)\", Default" "Color Presets" {
    tunnel: [w313 T23 {"DS5p- 1"=0.30136988, "colorCorrection 2"=-0.05479452, "colorCorrection 3"=1.9726027, "colorCorrection 4"=0.9041096, "colorCorrection 5"=-0.41095892, "colorCorrection 6"=-1.6438357, "colorCorrection 7"=0.63013697, "colorCorrection 8"=1.7534246, "colorCorrection 9"=1.5068493, "colorCorrection 10"=-2.0, "colorCorrection 11"=1.9726027, "colorCorrection 12"=-1.2876712} ("STColorCorrection") T11 {"colorCorrection 1"=1.339452, "colorCorrection 2"=0.045342464, "colorCorrection 3"=0.80136985, "colorCorrection 4"=0.19479452, "colorCorrection 5"=-1.2150685, "colorCorrection 6"=-0.9254795, "colorCorrection 7"=0.4671233, "colorCorrection 8"=1.3315068, "colorCorrection 9"=1.7899219, "colorCorrection 10"=-1.1794521, "colorCorrection 11"=0.0779452, "colorCorrection 12"=0.049178082} ("STColorCorrection") T11 {"colorCorrection 1"=0.21917808, "colorCorrection 2"=-0.1369863, "colorCorrection 3"=0.79452056, "colorCorrection 4"=0.69452053, "colorCorrection 5"=-0.28095892, "colorCorrection 6"=-1.7138357, "colorCorrection 7"=0.78013694, "colorCorrection 8"=1.4534247, "colorCorrection 9"=0.9368493, "colorCorrection 10"=-1.7, "colorCorrection 11"=1.6836027, "colorCorrection 12"=-0.8076712} ("STColorCorrection") T11 {"colorCorrection 1"=0.5479452, "colorCorrection 2"=0.32876712, "colorCorrection 3"=0.82191783, "colorCorrection 4"=0.10958904, "colorCorrection 5"=-0.4050685, "colorCorrection 6"=-1.5254794, "colorCorrection 7"=0.9571233, "colorCorrection 8"=0.89150685, "colorCorrection 9"=1.189922, "colorCorrection 10"=-0.47945204, "colorCorrection 11"=0.047945205, "colorCorrection 12"=-0.27082193} ("STColorCorrection") T11 {"colorCorrection 1"=0.5479452, "colorCorrection 2"=0.32876712, "colorCorrection 3"=0.37, "colorCorrection 4"=0.11958904, "colorCorrection 5"=-0.044, "colorCorrection 6"=-1.43, "colorCorrection 7"=0.707, "colorCorrection 8"=0.89050686, "colorCorrection 9"=0.766922, "colorCorrection 10"=-0.47945204, "colorCorrection 11"=0.2099452, "colorCorrection 12"=-0.28982192} ("STColorCorrection") w319 T11 {"colorCorrection 1"=-0.1369863, "colorCorrection 2"=1.3424658, "colorCorrection 3"=1.6986301, "colorCorrection 4"=1.7534246, "colorCorrection 5"=-0.8767123, "colorCorrection 6"=-1.9452055, "colorCorrection 7"=1.4520547, "colorCorrection 8"=1.5616438, "colorCorrection 9"=1.479452, "colorCorrection 10"=-2.0, "colorCorrection 11"=1.3972603, "colorCorrection 12"=-0.65753424} ("STColorCorrection") T11 {"colorCorrection 1"=0.30136988, "colorCorrection 2"=-0.05479452, "colorCorrection 3"=1.9726027, "colorCorrection 4"=0.9041096, "colorCorrection 5"=-0.7123288, "colorCorrection 6"=-2.0, "colorCorrection 7"=0.79452056, "colorCorrection 8"=1.99, "colorCorrection 9"=1.3468493, "colorCorrection 10"=-2.0, "colorCorrection 11"=1.8466027, "colorCorrection 12"=-1.3068492} ("STColorCorrection") T11 {"colorCorrection 1"=0.5479452, "colorCorrection 2"=0.32876712, "colorCorrection 3"=0.82191783, "colorCorrection 4"=0.10958904, "colorCorrection 5"=-0.4050685, "colorCorrection 6"=-1.5254794, "colorCorrection 7"=0.9571233, "colorCorrection 8"=0.89150685, "colorCorrection 9"=0.7671233, "colorCorrection 10"=-0.47945204, "colorCorrection 11"=0.047945205, "colorCorrection 12"=-0.27082193} ("STColorCorrection") T11 {"colorCorrection 1"=0.40136987, "colorCorrection 2"=0.047945205, "colorCorrection 3"=1.9178082, "colorCorrection 4"=0.5479452, "colorCorrection 5"=-1.5999494, "colorCorrection 6"=-0.48342466, "colorCorrection 7"=1.3093151, "colorCorrection 8"=0.79, "colorCorrection 9"=1.9508219, "colorCorrection 10"=-1.9952055, "colorCorrection 11"=0.87660265, "colorCorrection 12"=-0.7039726} ("STColorCorrection") w324 w325 w326 w327 w328 T11 {"colorCorrection 1"=0.5479452, "colorCorrection 2"=1.3701172, "colorCorrection 3"=0.65722656, "colorCorrection 4"=0.60253906, "colorCorrection 5"=1.99, "colorCorrection 6"=0.19178082, "colorCorrection 7"=-1.2602739, "colorCorrection 8"=-0.5751953, "colorCorrection 9"=-0.43835616, "colorCorrection 10"=0.24609375, "colorCorrection 11"=-0.7675781, "colorCorrection 12"=1.3154297} ("STColorCorrection") T11 {"colorCorrection 1"=0.12988281, "colorCorrection 2"=0.39941406, "colorCorrection 3"=0.39941406, "colorCorrection 4"=-0.06933594, "colorCorrection 5"=-0.19824219, "colorCorrection 6"=-0.4033203, "colorCorrection 7"=-0.4033203, "colorCorrection 8"=1.0058594, "colorCorrection 9"=0.921875, "colorCorrection 10"=-0.44140625, "colorCorrection 11"=-0.44140625, "colorCorrection 12"=-0.0390625} ("Read color")] -> w15
    tunnel: "STColorCorrection" -> [w313 _ _ _ _ _ _ _ _ _ _ _ _ _ _ _ _ _]
    frame "Custom" {
    }
    frame "RS400 (DS5p)", Default {
    }
    frame "RS400 (DS5p) 2" {
    }
    frame "RS400 (DS5p) 3" {
    }
    frame "RS400 (DS5p) 4" {
    }
    frame "RS400 (DS5p) 5" {
    }
    frame "RS410 (DS5a)" {
      w319 = T11 {"colorCorrection 1"=0.30136988, "colorCorrection 2"=-0.05479452, "colorCorrection 3"=1.9726027, "colorCorrection 4"=0.9041096, "colorCorrection 5"=-0.84931505, "colorCorrection 6"=-1.8082192, "colorCorrection 7"=1.3424658, "colorCorrection 8"=1.7808219, "colorCorrection 9"=1.5068493, "colorCorrection 10"=-2.0, "colorCorrection 11"=1.9726027, "colorCorrection 12"=-1.2876712}  # DS5p
    }
    frame "RS410 (DS5a) 2" {
    }
    frame "DS410 (DS5a) 3" {
    }
    frame "DS410 (DS5a) 4" {
    }
    frame "DS410+IR" {
    }
    frame "DS5LR" {
      w324 = T24 {"Color 0"=0.795, "Color 1"=0.71, "Color 2"=0.493, "Color 3"=0.11, "Color 4"=-0.329, "Color 5"=-1.5902739726027402, "Color 6"=1.1, "Color 7"=1.04, "Color 8"=1.01, "Color 9"=-0.479, "Color 10"=-0.164, "Color 11"=-0.274}  # DS5LR
    }
    frame "DS5LR-2" {
      w325 = T24 {"Color 0"=0.2988, "Color 1"=0.2939, "Color 2"=0.2939, "Color 3"=0.114, "Color 4"=-0.1689, "Color 5"=-0.0849, "Color 6"=-0.0849, "Color 7"=0.5, "Color 8"=0.5, "Color 9"=-0.148, "Color 10"=-0.2109, "Color 11"=-0.081}  # DS5LR1
    }
    frame "DS5LR no pattern" {
      w326 = T24 {"Color 0"=1.9178082191780819, "Color 1"=1.99, "Color 2"=-2.0, "Color 3"=-2.0, "Color 4"=-1.041095890410959, "Color 5"=0.05479452054794498, "Color 6"=-0.2191780821917808, "Color 7"=0.904109589041096, "Color 8"=0.904109589041096, "Color 9"=-0.547945205479452, "Color 10"=-0.13698630136986312, "Color 11"=-0.19178082191780832}  # DS5LR no IR pattern
    }
    frame "RS410 Remove IR" {
      w327 = T24 {"Color 0"=0.4384765625, "Color 1"=1.990234375, "Color 2"=1.990234375, "Color 3"=-2.0, "Color 4"=-1.83984375, "Color 5"=-0.21875, "Color 6"=1.009765625, "Color 7"=1.33984375, "Color 8"=1.73046875, "Color 9"=-1.9951171875, "Color 10"=0.5751953125, "Color 11"=-0.4931640625}  # DS5 no pattern
    }
    frame "RS410 Remove IR 2" {
      w328 = T24 {"Color 0"=0.5205479452054793, "Color 1"=1.99, "Color 2"=1.506849315068493, "Color 3"=-2.0, "Color 4"=-2.0, "Color 5"=-0.08219178082191791, "Color 6"=1.1232876712328768, "Color 7"=1.013698630136986, "Color 8"=1.698630136986301, "Color 9"=-2.0, "Color 10"=0.5753424657534243, "Color 11"=-0.41095890410958913}  # No pattern 3
    }
    frame "DS5micro" {
      (unwired) T11 {"colorCorrection 1"=1.3424658, "colorCorrection 2"=1.369863, "colorCorrection 3"=0.65753424, "colorCorrection 4"=0.60273975, "colorCorrection 5"=1.2876712, "colorCorrection 6"=-0.10958904, "colorCorrection 7"=-0.5753425, "colorCorrection 8"=-0.5753425, "colorCorrection 9"=-1.0410959, "colorCorrection 10"=0.24657534, "colorCorrection 11"=-0.7671233, "colorCorrection 12"=1.3150685} ("STColorCorrection 2")
      (unwired) T11 {"colorCorrection 1"=1.150685, "colorCorrection 2"=1.5068493, "colorCorrection 3"=1.6164384, "colorCorrection 4"=0.08219178, "colorCorrection 5"=1.99, "colorCorrection 6"=-0.7671233, "colorCorrection 7"=-0.82191783, "colorCorrection 8"=-0.60273975, "colorCorrection 9"=0.10958904, "colorCorrection 10"=0.19178082, "colorCorrection 11"=-1.369863, "colorCorrection 12"=1.9452055} ("STColorCorrection")
    }
    frame "D435" {
    }
  }
  n13 = call "rs3 Advanced Set Census Enable Reg3.vi"("error in (no error)"="error in (no error)", "ST_CensusEnableReg"=w21, "device in"="device in") -> ("error out 2"=w89:errorcluster, "error"=w58:u64, "Dev out"=w88:u64)  [unwired: 6 in]
  n14 = call "rs3 Advanced AE setpoint3.vi"("error in (no error)"=w89, "ST_AE_Control"=w19, "device in"=w88) -> ("error out"=w87:errorcluster, "error"=w56:u64, "Dev out"=w86:u64)  [unwired: 6 in]
  n15 = call "rs3 Advanced set depth table control3.vi"("error in (no error)"=w87, "Depth Table"=w17, "device in"=w86) -> ("error out 2"=w85:errorcluster, "error"=w54:u64, "Dev out"=w84:u64)  [unwired: 6 in]
  n16 = call "rs3 Advanced set depth control3.vi"("error in (no error)"=w85, "depth control"=w63, "device in"=w84) -> ("error out"=w83:errorcluster, "error"=w52:u64, "Dev out"=w82:u64)  [unwired: 6 in]
  n17 = call "rs3 Advanced set HDAD3.vi"("error in (no error)"=w83, "HDAD"=w61, "device in"=w82) -> ("error out"=w81:errorcluster, "error"=w51:u64, "Dev out"=w80:u64)  [unwired: 6 in]
  n18 = call "rs3 Advanced set SLO Penalty3.vi"("error in (no error)"=w81, "ST SLO Penalty"=w33, "device in"=w80) -> ("error out"=w79:errorcluster, "error"=w50:u64, "Dev out"=w78:u64)  [unwired: 6 in]
  n19 = call "rs3 Advanced set SLO Threshold3.vi"("error in (no error)"=w79, "ST SLO Threshold"=w30, "device in"=w78) -> ("error out"=w77:errorcluster, "error"=w49:u64, "Dev out"=w76:u64)  [unwired: 6 in]
  n20 = call "rs3 Advanced set RAU control3.vi"("error in (no error)"=w77, "ST RAU vector"=w27, "device in"=w76) -> ("error out"=w75:errorcluster, "error"=w48:u64, "Dev out"=w74:u64)  [unwired: 6 in]
  n21 = call "rs3 Advanced set Rau Threshold3.vi"("error in (no error)"=w75, "ST Rau Threshold"=w28, "device in"=w74) -> ("error out"=w73:errorcluster, "error"=w47:u64, "Dev out"=w72:u64)  [unwired: 6 in]
  n22 = case shown="True" "Set Color Corr" {
    tunnel: w73 -> [w332 w339]
    tunnel: w72 -> [w333 w338]
    tunnel: w15 -> [_ w337]
    tunnel: [w332 w336] -> w71
    tunnel: [w333 w335] -> w70
    tunnel: [u64 0 ("error") w334] -> w45
    frame False {
    }
    frame True {
      n23 = call "rs3 Advanced set color correction3.vi"("error in (no error)"=w339, "STColorCorrection input"=w337, "device in"=w338) -> ("error out"=w336:errorcluster, "error"=w334:u64, "Dev out"=w335:u64)  [unwired: 6 in]
    }
  }
  n24 = call "rs3 Advanced set Color control3.vi"("error in (no error)"=w71, "ST Color Control"=w23, "device in"=w70) -> ("error out"=w69:errorcluster, "error"=w44:u64, "Dev out"=w68:u64)  [unwired: 6 in]
  n25 = call "rs3 Advanced set RSM control3.vi"("error in (no error)"=w69, "ST RSM"=w25, "device in"=w68) -> ("error out"=w1:errorcluster, "error"=w46:u64, "Dev out"=→"Dev out":u64)  [unwired: 6 in]
  n26 = call "rs3 showError.vi"("error in (no error)"=w1, "error"=w58) -> ("error out"=w13:errorcluster, "Error summary"=w57:string)  [unwired: 5 in, 3 out]
  n27 = call "rs3 showError.vi"("error in (no error)"=w13, "error"=w56) -> ("error out"=w12:errorcluster, "Error summary"=w55:string)  [unwired: 5 in, 3 out]
  n28 = call "rs3 showError.vi"("error in (no error)"=w12, "error"=w54) -> ("error out"=w11:errorcluster, "Error summary"=w53:string)  [unwired: 5 in, 3 out]
  n29 = call "rs3 showError.vi"("error in (no error)"=w11, "error"=w52) -> ("error out"=w10:errorcluster, "Error summary"=w43:string)  [unwired: 5 in, 3 out]
  n30 = call "rs3 showError.vi"("error in (no error)"=w10, "error"=w51) -> ("error out"=w9:errorcluster, "Error summary"=w42:string)  [unwired: 5 in, 3 out]
  n31 = call "rs3 showError.vi"("error in (no error)"=w9, "error"=w50) -> ("error out"=w8:errorcluster, "Error summary"=w41:string)  [unwired: 5 in, 3 out]
  n32 = call "rs3 showError.vi"("error in (no error)"=w8, "error"=w49) -> ("error out"=w7:errorcluster, "Error summary"=w40:string)  [unwired: 5 in, 3 out]
  n33 = call "rs3 showError.vi"("error in (no error)"=w7, "error"=w48) -> ("error out"=w6:errorcluster, "Error summary"=w39:string)  [unwired: 5 in, 3 out]
  n34 = call "rs3 showError.vi"("error in (no error)"=w6, "error"=w46) -> ("error out"=w5:errorcluster, "Error summary"=w60:string)  [unwired: 5 in, 3 out]
  n35 = call "rs3 showError.vi"("error in (no error)"=w5, "error"=w47) -> ("error out"=w4:errorcluster, "Error summary"=w38:string)  [unwired: 5 in, 3 out]
  n36 = call "rs3 showError.vi"("error in (no error)"=w4, "error"=w45) -> ("error out"=w3:errorcluster, "Error summary"=w37:string)  [unwired: 5 in, 3 out]
  n37 = call "rs3 showError.vi"("error in (no error)"=w3, "error"=w44) -> ("error out"=→"error out":errorcluster, "Error summary"=w35:string)  [unwired: 5 in, 3 out]
  n38 = Concatenate Strings(w57, w36, w55, w36, w53, w36, w43, w36, w42, w36, w41, w36, w40, w36, w39, w36, w60, w36, w38, w36, w37, w36, w35) -> (→"Set advanced error":string)
